vi "SMC_GetSwSt.vi"(8 "error in (no error)":errorcluster) -> (0 "error out":errorcluster, 1 "Switches Max":bool[](array[boolean]), 3 "Switches Min":bool[](array[boolean]))   [LabVIEW 2015]
uses:
  SMC_SubVIs.llb/SMC_ManagerMode.ctl
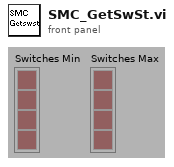
[diagram p1: front panel]
types:
  T1 = typedef "SMC_ManagerMode.ctl" = enum16{"Init", "Get", "SetPosition", "SetStatus", "SetMoving", "SetControllerNr"}
  T2 = typedef "SMC Paras.ctl" = cluster{"VENUS Language":T3, "Number of Axis":u8, "Controller Nr":u8, "Simulation":bool}
  T3 = typedef "VENUSNr.ctl" = enum16{"VENUS 2", "VENUS 1"}
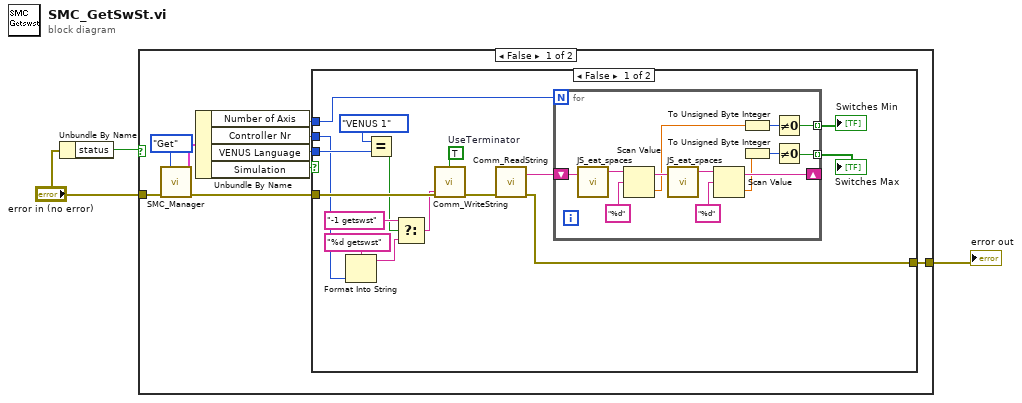
[diagram p0: block diagram]
diagram:
  n1 = Unbundle By Name("error in (no error)") -> ("status"=w3:bool)
  n2 = case shown="False" w3 {
    tunnel: "error in (no error)" -> [w11 w43]
    tunnel: [w9 w43] -> w1
    frame False {
      n3 = call "SMC_Manager.vi"("Mode"=SMC_ManagerMode."Get", "error in (no error)"=w11) -> ("SMC Parameter Out"=w8:T2, "error out"=w10:errorcluster)  [unwired: 9 in, 3 out]
      n4 = Unbundle By Name(w8) -> ("Number of Axis"=w5:u8, "Controller Nr"=w6:u8, "VENUS Language"=w7:T3, "Simulation"=w4:bool)
      n5 = case shown="False" w4 {
        tunnel: w10 -> [w25 w42]
        tunnel: [w23 w42] -> w9
        tunnel: w7 -> [w21 _]
        tunnel: w6 -> [w15 _]
        tunnel: w5 -> [w14 _]
        frame False {
          w13 = TRUE  # UseTerminator
          n6 = Format Into String(format string="%d getswst" ("Format String"), w15) -> (resulting string=w17:string)  [unwired: 2 in, 1 out]
          n7 = Equal?(x=enum16{"VENUS 2", "VENUS 1"}."VENUS 1", y=w21) -> (x = y?=w16:bool)
          n8 = Select(t="-1 getswst" ("Substring"), s=w16, f=w17) -> (s? t:f=w20:string)
          n9 = call "Comm_WriteString.vi"("string to write"=w20, "error in (no error)"=w25, "UseTerminator"=w13) -> ("error out"=w24:errorcluster)  [unwired: 8 in]
          n10 = call "Comm_ReadString.vi"("error in (no error)"=w24) -> ("error out"=w23:errorcluster, "Answer"=w28:string)  [unwired: 9 in]
          n11 = for {
            N: w14 -> [_]
            tunnel: [w31] -> w26 mode=indexing
            tunnel: [w29] -> w27 mode=indexing
            shift-right: [w35] -> _
            shift-left: w28 -> [w36]
            n12 = call "JS_eat_spaces.vi"("String In"=w36) -> ("String Out"=w40:string)
            n13 = Scan Value(string=w40, format string="%d" ("Format-String")) -> (output string=w38:string, value=w34:dbl)  [unwired: 1 in]
            n14 = call "JS_eat_spaces.vi"("String In"=w38) -> ("String Out"=w37:string)
            n15 = Scan Value(string=w37, format string="%d" ("Format-String")) -> (output string=w35:string, value=w33:dbl)  [unwired: 1 in]
            n16 = To Unsigned Byte Integer(number=w34) -> (unsigned 8bit integer=w32:u8)
            n17 = To Unsigned Byte Integer(number=w33) -> (unsigned 8bit integer=w30:u8)
            n18 = Not Equal To 0?(x=w32) -> (x != 0?=w31:bool)
            n19 = Not Equal To 0?(x=w30) -> (x != 0?=w29:bool)
          }
          "Switches Min" <- w26
          "Switches Max" <- w27
        }
        frame True {
          # "Simulation"
        }
      }
    }
    frame True {
      # "Error, do nothing"
    }
  }
  "error out" <- w1
